vi "AlliGator Remove Duplicated Fit Parameter Constraints.vi"(8 "Error In":errorcluster, 9 "New Constraints in":T1[](array[typedef]) {"Max Value" format="%#.3g"; "Min Value" format="%#.3g"}, 11 "Old Constraints":T1[](array[typedef]) {"Max Value" format="%#.3g"; "Min Value" format="%#.3g"}) -> (0 "Error Out":errorcluster, 3 "New Constraints out":T1[](array[typedef]) {"Max Value" format="%#.3g"; "Min Value" format="%#.3g"})   [LabVIEW 2021, in "AlliGator Settings.lvlib"]
doc: "Removes any potential duplicate entries in the array of fit parameter constraints."
uses:
  AlliGator Settings.lvlib
  AlliGator Decay Fit Parameter Constraints 2.ctl
  Fits/IRF(X)PSED/Decay Fit Parameters In List.ctl
  359a0e18-36cc-47c1-bd4d-14aca24d9214.vi
  462271ff-30ec-4d38-93df-9dde4097cd5c.vi
  359a0e18-36cc-47c1-bd4d-14aca24d9214.vi/8dd81a27-1ff4-4680-915d-7458584d3105.vi
  <userlib>/_OpenG.lib/array/array.llb/Sort Array__ogtk.vi
  <userlib>/_OpenG.lib/array/array.llb/Sort 1D Array (I32)__ogtk.vi
  <userlib>/_OpenG.lib/array/array.llb/Reorder Array2__ogtk.vi
  <userlib>/_OpenG.lib/array/array.llb/Reorder 1D Array2 (I32)__ogtk.vi
  <userlib>/_OpenG.lib/array/array.llb/Delete Elements from 1D Array (Variant)__ogtk.vi
  <userlib>/_OpenG.lib/array/array.llb/openg_array.lvlib
  AlliGator Decay Fit.lvlib
  Fits/Fits.lvlib
panel:
  # "see the AlliGator License on the block diagram (Ctrl+E or Window:Show Block Diagram)"
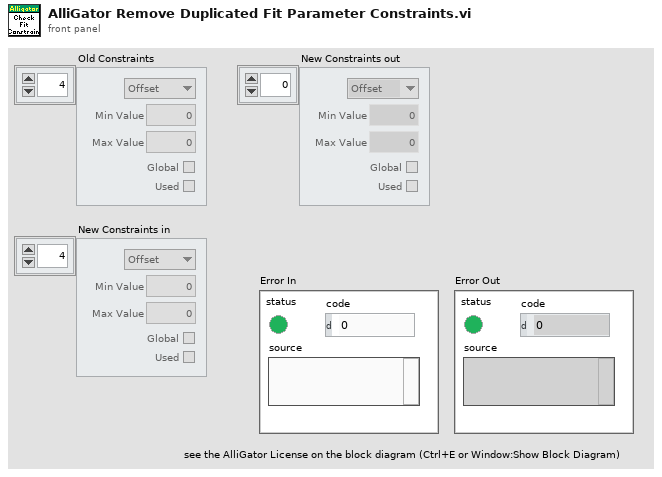
[diagram p1: front panel]
types:
  T1 = typedef "AlliGator Decay Analysis.lvlib/AlliGator Decay Fit.lvlib/AlliGator Decay Fit Parameter Constraints 2.ctl" = cluster{"Fit Parameter":T2, "Min Value":dbl, "Max Value":dbl, "Global":bool, "Used":bool}
  T2 = typedef "Fits.lvlib/Decay Fit Parameters In List.ctl" = enum16{"Offset", "Baseline", "A_1", "tau_1", "A_2", "tau_2"}
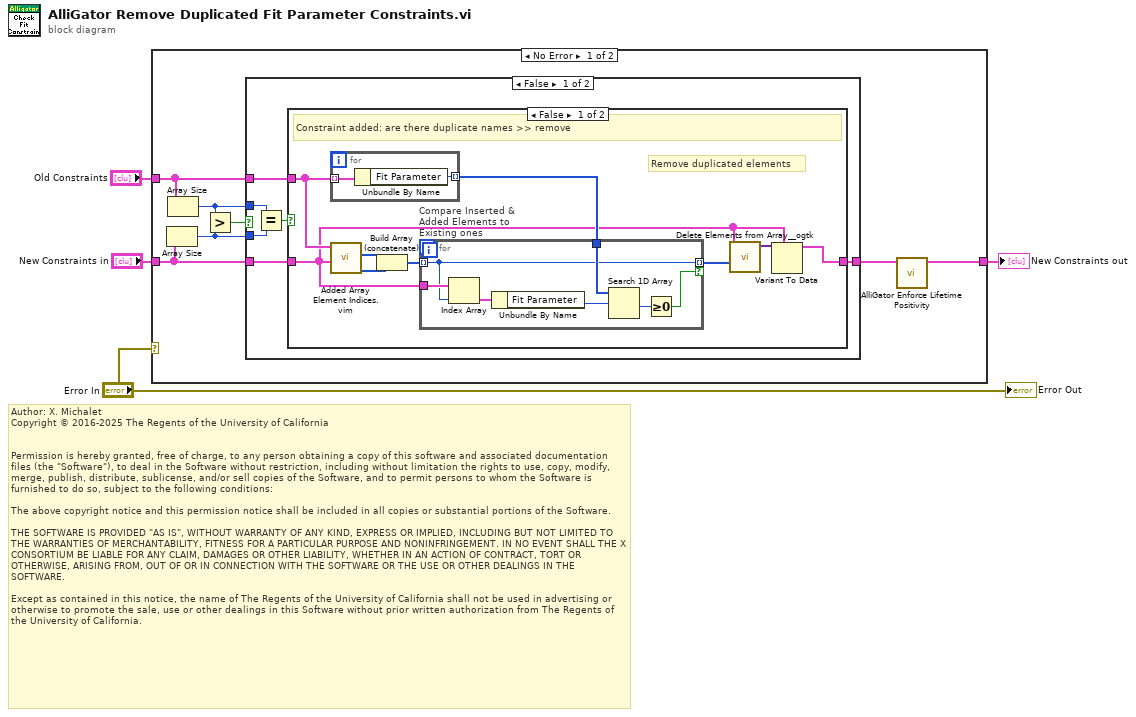
[diagram p0: block diagram]
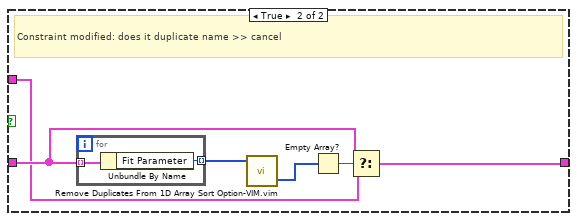
[diagram p2: hidden frame]
diagram:
  # "Author: X. Michalet\nCopyright © 2016-2025 The Regents of the University of California\n \n\nPermission is hereby granted, free of charge, to any person obtaining a copy of this software and associated documentation files (the \"Software\"), to deal in the Software without restriction, including without limitation the rights to use, copy, modify, merge, publish, distribute, sublicense, and/or sell copies of the Software, and to permit persons to whom the Software is furnished to do so, subject to the following conditions:\n\nThe above copyright notice and this permission notice shall be included in all copies or substantial portions of the Software.\n\nTHE SOFTWARE IS PROVIDED \"AS IS\", WITHOUT WARRANTY OF ANY KIND, EXPRESS OR IMPLIED, INCLUDING BUT NOT LIMITED TO THE WARRANTIES OF MERCHANTABILITY, FITNESS FOR A PARTICULAR PURPOSE AND NONINFRINGEMENT. IN NO EVENT SHALL THE X CONSORTIUM BE LIABLE FOR ANY CLAIM, DAMAGES OR OTHER LIABILITY, WHETHER IN AN ACTION OF CONTRACT, TORT OR OTHERWISE, ARISING FROM, OUT OF OR IN CONNECTION WITH THE SOFTWARE OR THE USE OR OTHER DEALINGS IN THE SOFTWARE.\n\nExcept as contained in this notice, the name of The Regents of the University of California shall not be used in advertising or otherwise to promote the sale, use or other dealings in this Software without prior written authorization from The Regents of the University of California."
  n1 = case shown="No Error" "Error In" {
    tunnel: "New Constraints in" -> [w10 w45]
    tunnel: [w5 w45] -> w3
    tunnel: "Old Constraints" -> [w8 _]
    frame No Error {
      n2 = Array Size(array=w10) -> (size(s)=w7:i32)
      n3 = Array Size(array=w8) -> (size(s)=w6:i32)
      n4 = Greater?(x=w6, y=w7) -> (0:w11:bool)
      n5 = case shown="False" w11 {
        tunnel: w10 -> [w13 w44]
        tunnel: [w12 w44] -> w9
        tunnel: w8 -> [w14 _]
        tunnel: w7 -> [w16 _]
        tunnel: w6 -> [w17 _]
        frame False {
          n6 = Equal?(x=w17, y=w16) -> (x = y?=w15:bool)
          n7 = case shown="False" w15 {
            tunnel: w14 -> [w26 w39]
            tunnel: w13 -> [w22 w41]
            tunnel: [w20 w40] -> w12
            frame False {
              # "Remove duplicated elements"
              # "Constraint added: are there duplicate names >> remove"
              n8 = for {
                tunnel: w26 -> [w35] mode=indexing
                tunnel: [w34] -> w24 mode=indexing
                n9 = Unbundle By Name(w35) -> ("Fit Parameter"=w34:T2)
              }
              n10 = call "Added Array Element Indices.vim"("New Array"=w22, "Old Array"=w26) -> ("Appended Element Indices in New Array"=w18:i32[], "Inserted Element Indices in New Array"=w19:i32[])  [unwired: 6 in, 2 out]
              n11 = Build Array (concatenate)(w19, w18) -> (w25:i32[])
              n12 = for "Compare Inserted & Added Elements to Existing ones" {
                tunnel: w25 -> [w28] mode=indexing
                tunnel: w22 -> [w33]
                tunnel: w24 -> [w31]
                tunnel: [w28] -> w23 mode=indexing if=w27
                n13 = Index Array(array=w33, index=w28) -> (element=w32:T1)
                n14 = Unbundle By Name(w32) -> ("Fit Parameter"=w30:T2)
                n15 = Search 1D Array(1D array=w31, element=w30) -> (index of element=w29:i32)  [unwired: 1 in]
                n16 = Greater Or Equal To 0?(x=w29) -> (x >= 0?=w27:bool)
              }
              n17 = call-poly <userlib>:"Delete Elements from Array__ogtk.vi"("indices"=w23, "array"=w22) -> ("array w/ subset deleted"=w21:variant[])  [unwired: 8 in, 1 out]
              n18 = Variant To Data(type=w22, Variant=w21) -> (data=w20:T1[])  [unwired: 1 in, 1 out]
            }
            frame True {
              # "Constraint modified: does it duplicate name >> cancel"
              n19 = for {
                tunnel: w41 -> [w43] mode=indexing
                tunnel: [w42] -> w38 mode=indexing
                n20 = Unbundle By Name(w43) -> ("Fit Parameter"=w42:T2)
              }
              n21 = call "Remove Duplicates From 1D Array Sort Option-VIM.vim"("Input Array"=w38) -> ("Indices of Removed Elements"=w37:i32[])  [unwired: 1 in, 1 out]
              n22 = Empty Array?(array=w37) -> (empty?=w36:bool)
              n23 = Select(t=w41, s=w36, f=w39) -> (s? t:f=w40:T1[])
            }
          }
        }
        frame True {
          # "Constraint deleted: no checks"
        }
      }
      n24 = call "AlliGator Enforce Lifetime Positivity.vi"("Constraints in"=w9) -> ("Constraints out"=w5:T1[])  [unwired: 10 in]
    }
    frame Error {
    }
  }
  "New Constraints out" <- w3
  "Error Out" <- "Error In"
